vi "Tracepoint_BurstModeComplete.vi"(5 "new count":i32, 7 "prev count":i32, 8 "error in (no error)":errorcluster, 9 "group":string, 10 "type":string, 11 "Qbus":refnum<class "Qbus.lvclass">) -> (0 "error out":errorcluster, 3 "Qbus out":refnum<class "Qbus.lvclass">)   [LabVIEW 2017, in "BurstMode.lvlib"]
uses:
  <vilib>/addons/InsightCM/Devices/Shared/Cms/CmsBurstMode/BurstMode.lvlib
  <vilib>/addons/Qbus/Qbus.lvclass
  <vilib>/addons/TraceLogger/TraceLogger.lvlib
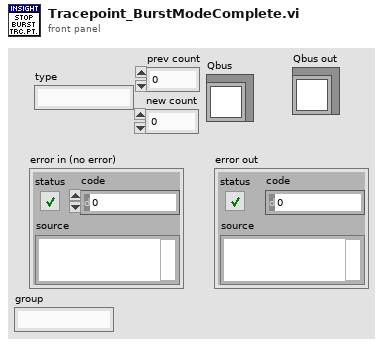
[diagram p1: front panel]
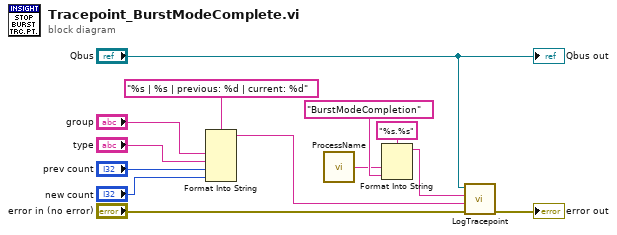
[diagram p0: block diagram]
diagram:
  n1 = Format Into String(format string="%s | %s | previous: %d | current: %d", "group", "type", "prev count", "new count") -> (resulting string=w8:string)  [unwired: 2 in, 1 out]
  n2 = call <vilib>:"ProcessName.vi"() -> ("process name"=w6:string)  [unwired: 5 in]
  n3 = Format Into String(format string="%s.%s", w6, "BurstModeCompletion" ("tracepoint")) -> (resulting string=w9:string)  [unwired: 2 in, 1 out]
  n4 = call <vilib>:"LogTracepoint.vi"("error in (no error)"="error in (no error)", "log string"=w8, "tracepoint"=w9, "qbus in"="Qbus") -> ("error out"=→"error out":errorcluster)  [unwired: 6 in, 1 out]
  "Qbus out" <- "Qbus"
